vi "configuration UI.vi"() -> ()   [LabVIEW 2013, in "Shared Memory Editor Node.lvclass"]
doc: "Copyright 2016 National Instruments Corporation\n\nLicensed under the Apache License, Version 2.0 (the \"License\"); you may not use this file except in compliance with the License. You may obtain a copy of the License at http://www.apache.org/licenses/LICENSE-2.0\nUnless required by applicable law or agreed to in writing, software distributed under the License is distributed on an \"AS IS\" BASIS, WITHOUT WARRANTIES OR CONDITIONS OF ANY KIND, either express or implied. See the License for the specific language governing permissions and limitations under the License."
uses:
  Shared Memory Editor Node.lvclass
  <vilib>/NI/DCAF UI Toolkit/Controls/Remove.ctl
  <vilib>/NI/DCAF UI Toolkit/Controls/Add.ctl
  <vilib>/NI/Configuration Framework/Node/NodeRef.ctl
  <vilib>/NI/Configuration Framework/Node/NISE_CEF_Node.lvclass
  <vilib>/NI/AMC/Message Queue.ctl
  <vilib>/NI/AMC/Message.ctl
  <vilib>/NI/Tools/Keyed Array/KeyedArray.ctl
  <vilib>/NI/Configuration Framework/Node/UserEventRef.ctl
  <vilib>/NI/Configuration Framework/Controls/EventCluster.ctl
  <vilib>/NI/Configuration Framework/Node/StopEvent.ctl
  <vilib>/NI/Configuration Framework/Node/RefreshUIEvent.ctl
  <vilib>/NI/Configuration Framework/Node/CacheState.ctl
  <vilib>/NI/Configuration Framework/Node/NodeChangeEvent.ctl
  <vilib>/NI/Tag Bus/tag/Data Type.ctl
  <vilib>/NI/DCAF/Tag Editor Core/control module/editor node/channel action event.ctl
  <vilib>/NI/DCAF/Tag Editor Core/control module/editor node/dialog output action.ctl
  <vilib>/NI/Tag Bus Module Framework/channel/TBM channel.lvclass
  <vilib>/NI/Tag Bus/tag/tag descriptor.lvclass
  access.ctl
  <vilib>/NI/DCAF Table API/Table Manager/object ref.ctl
  <vilib>/NI/DCAF/Tag Editor Core/Configuration Editor/Classes/Engine Parent/Engine Parent Editor Node.lvclass
  <vilib>/NI/DCAF/Tag Editor Core/Configuration Editor/Classes/Module editor node/module editor node.lvclass
  <vilib>/NI/DCAF Table API/Table Manager/references.ctl
  <vilib>/NI/DCAF Table API/Listbox/Multi Column Listbox.lvclass
  <vilib>/Utility/miscctls.llb/LVPositionTypeDef.ctl
  <vilib>/NI/DCAF Table API/Listbox/Multi Column Listbox.lvclass/Multi Column Listbox.ctl
  <vilib>/NI/DCAF Table API/Table Manager/Table Manager.lvclass/Table Manager.ctl
  <vilib>/NI/DCAF Table API/Listbox/Write Listbox.vi
  <vilib>/NI/DCAF Table API/Table Manager/Write Top VI.vi
  <vilib>/NI/DCAF/Tag Editor Core/Configuration Editor/Classes/Engine Parent/read engine configuration.vi
  <vilib>/NI/Module Execution Interface/Engine Configuration/engine configuration.lvclass
  <vilib>/NI/DCAF/Tag Editor Core/control module/editor node/control module editor.lvclass
  <vilib>/NI/DCAF Table API/Table Manager/Table Manager.lvclass
  <vilib>/NI/Tools/Keyed Array/Tools_KeyedArray.lvlib
  <vilib>/NI/AMC/AMC.lvlib
  <vilib>/NI/Configuration Framework/NISE_CEF_TreeControl.lvlib
  <vilib>/NI/DCAF UI Toolkit/Controls/DCAF UI Elements.lvlib
panel:
  in  "data type":T1
  in  "access":T2
  in  "Top Level Tab Control":enum32{"<Main Page>", "Configuration"}(tab)
  in  "tag list box":i32(listbox)=1
  in  "remove tag":T3
  in  "Add tag":T4
  in  "write directory":string
  in  "read directory":string
  in  "user event out":refnum<user-event>
  in  "node change":T5
  in  "cache state":T6
  in  "refresh UI":T7
  in  "stop event":T8
  in  "user event":T9
  in  "main queue":T10
  in  "node ref":T11
  # "Directories relative to engine root (/dev/shm/<EngineName>)"
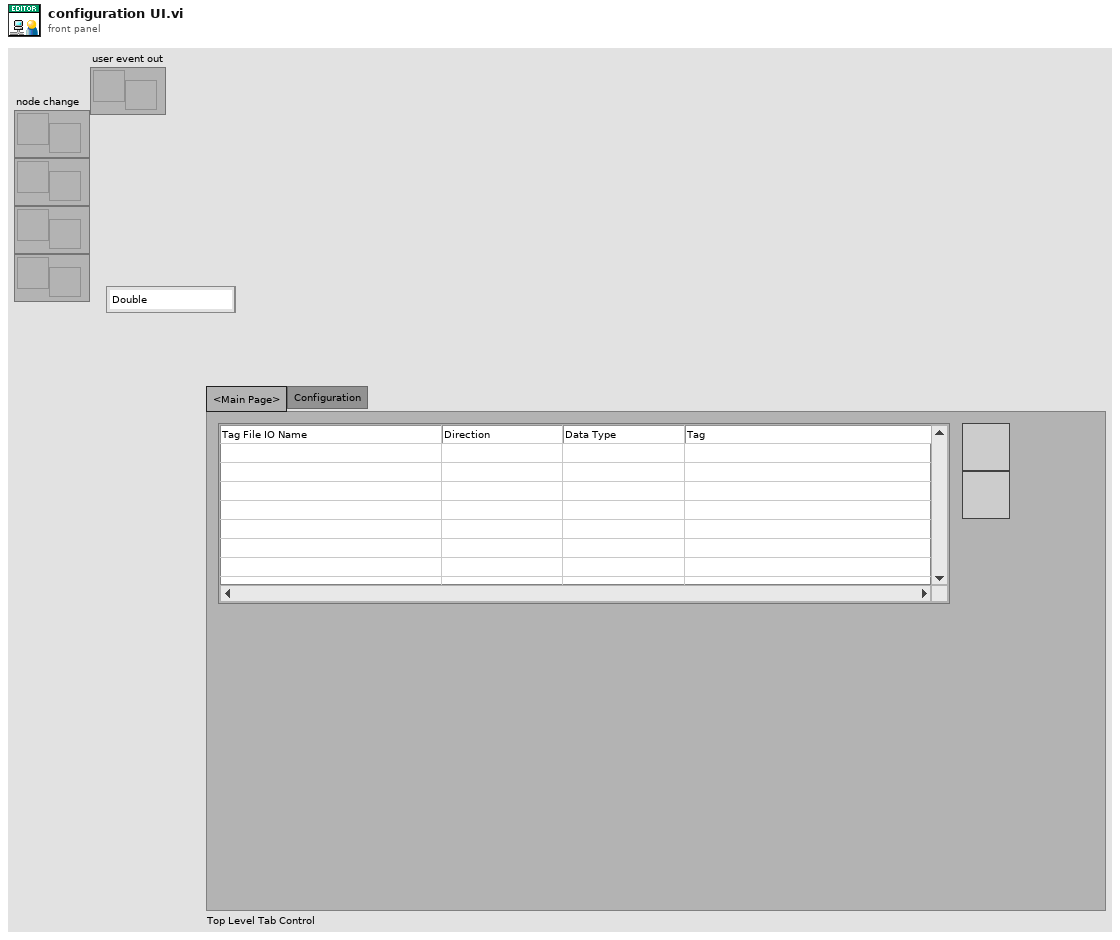
[diagram p1: front panel]
types:
  T1 = typedef "tag bus.lvlib/tag descriptor.lvclass/Data Type.ctl" = enum16{"Double", "Single", "I64", "I32", "I16", "I8", "U64", "U32", "U16", "U8", "Boolean", "String", "Array of Double", "Array of Single", "Array of I64", "Array of I32", "Array of I16", "Array of I8", "Array of U64", "Array of U32", "Array of U16", "Array of U8", "Array of Boolean", "Array of String"}
  T2 = typedef "Shared Memory Editor Node.lvclass/access.ctl" = enum16{"Read from File", "Write to File"}
  T3 = typedef "DCAF UI Elements.lvlib/Remove.ctl" = bool
  T4 = typedef "DCAF UI Elements.lvlib/Add.ctl" = bool
  T5 = typedef "NISE_CEF_Node.lvclass/NodeChangeEvent.ctl" = refnum<user-event>
  T6 = typedef "NISE_CEF_Node.lvclass/CacheState.ctl" = refnum<user-event>
  T7 = typedef "NISE_CEF_Node.lvclass/RefreshUIEvent.ctl" = refnum<user-event>
  T8 = typedef "NISE_CEF_Node.lvclass/StopEvent.ctl" = refnum<user-event>
  T9 = typedef "NISE_CEF_Node.lvclass/UserEventRef.ctl" = refnum<user-event>
  T10 = typedef "AMC.lvlib/Message Queue.ctl" = refnum<queue>
  T11 = typedef "NISE_CEF_Node.lvclass/NodeRef.ctl" = refnum<data-value>
  T12 = typedef "LVPositionTypeDef.ctl" = cluster{"Left":i32, "Top":i32}
  T13 = typedef "Table Manager.lvlib/Table Manager.lvclass/references.ctl" = cluster{"stop event":T8, "refresh UI":T7, "cache state":T6, "node change":T5, "user event out":refnum<user-event>, "main queue":T10, "user event":T9}
  T14 = typedef "Table Manager.lvlib/Table Manager.lvclass/object ref.ctl" = cluster{"engine":refnum<data-value>, "Node Ref":refnum<data-value>}
  T15 = typedef "Table Manager.lvlib/Column.lvclass/Column Descriptor.ctl" = cluster{"name":string, "caption":string, "Column Type":T16, "Params":string, "AutoSizeMode":i32, "FillWeight":sgl, "MinWidth":u32, "tooltip":string, "Enum Reference":refnum<vi>, "Channel suffix":string, "Read Only":bool, "Call Back VI":T17, "DT Dependency":i32, "name dependency":i32, "data type":T1}
  T16 = typedef "Table Manager.lvlib/Column.lvclass/Column Type.ctl" = enum16{"String", "Mapping", "Channel Name", "Tag", "Enum", "Data Type", "Numeric"}
  T17 = typedef "Table Manager.lvlib/Table Manager.lvclass/Call Back Ref Type Def.ctl" = refnum<vi>
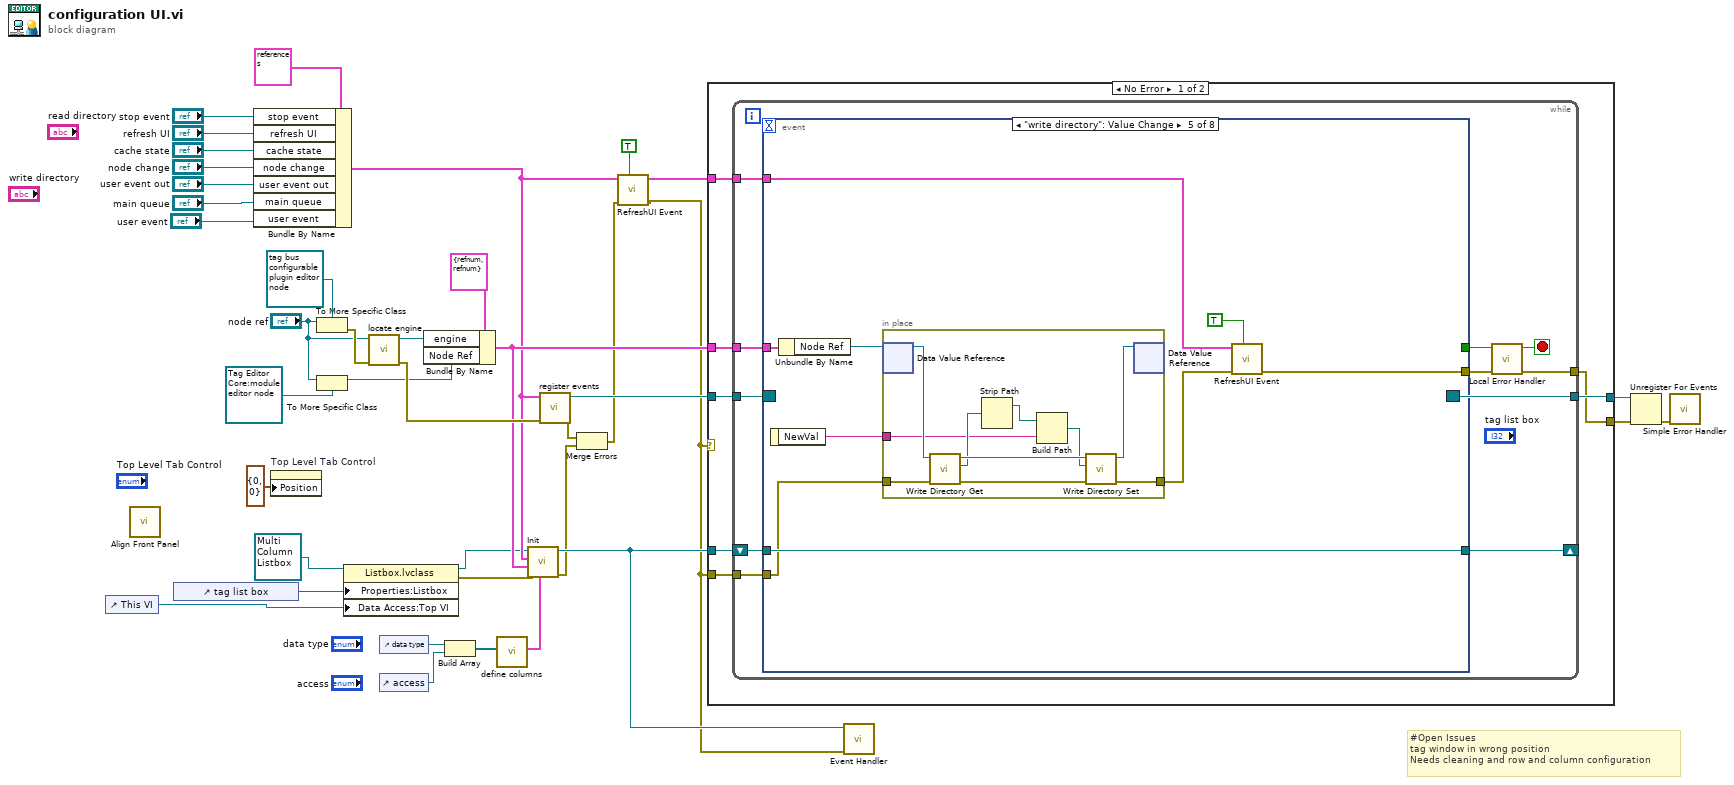
[diagram p0: block diagram]
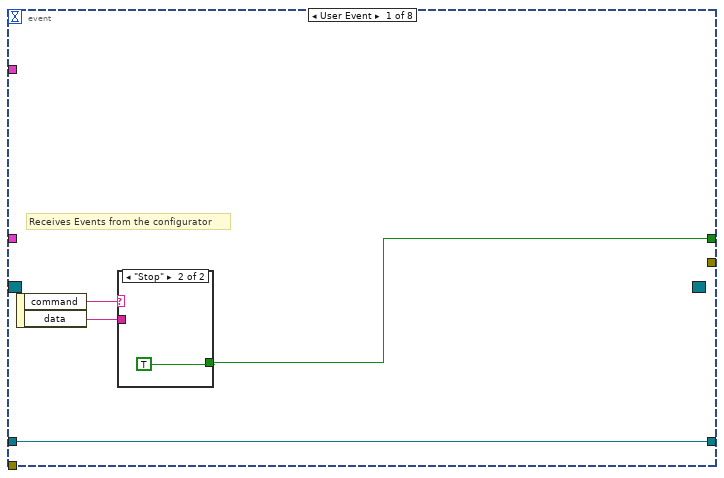
[diagram p2: hidden frame]
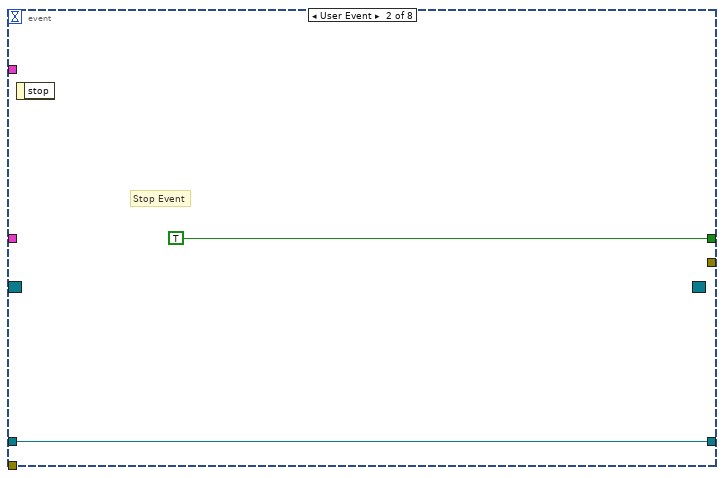
[diagram p4: hidden frame]
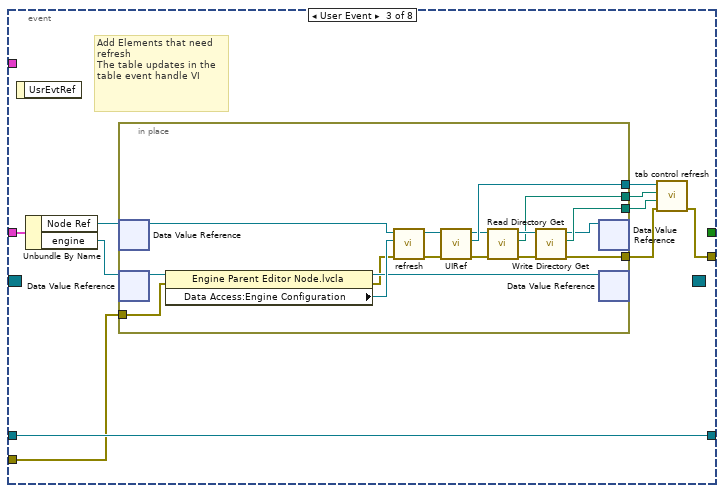
[diagram p5: hidden frame]
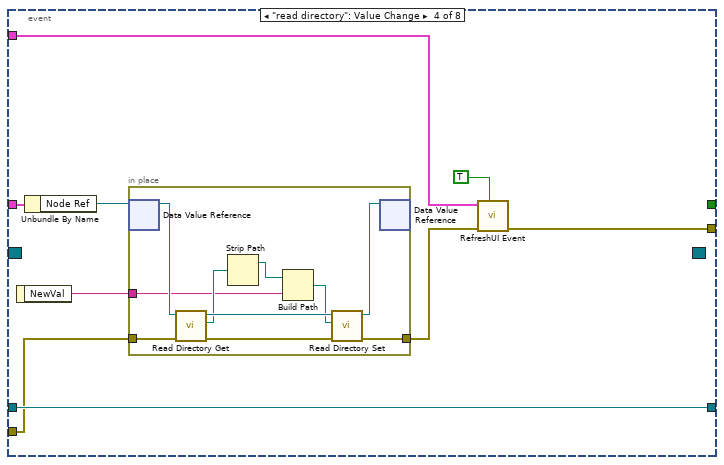
[diagram p6: hidden frame]
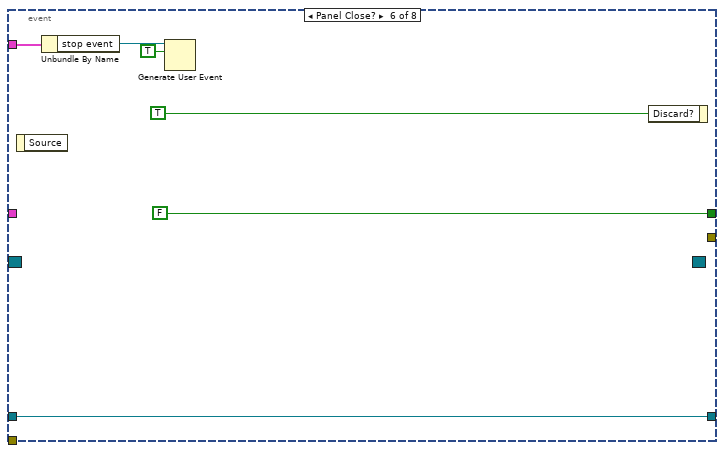
[diagram p7: hidden frame]
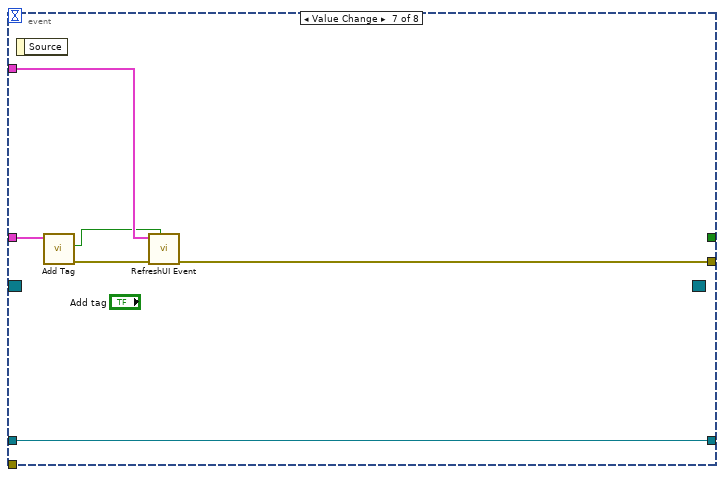
[diagram p8: hidden frame]
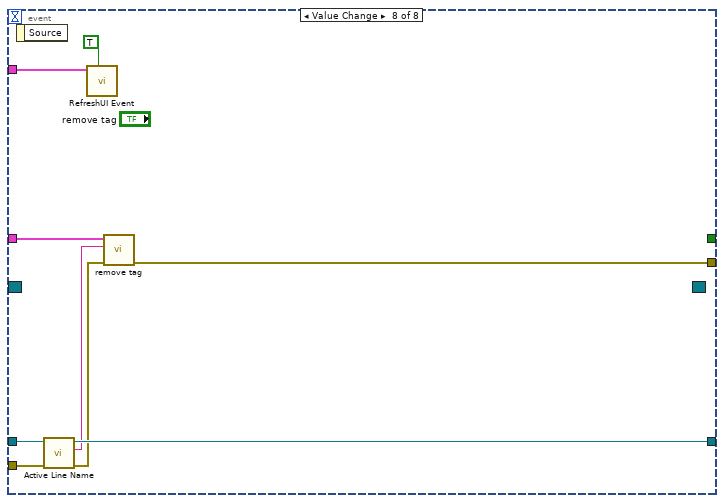
[diagram p9: hidden frame]
diagram:
  # "#Open Issues \ntag window in wrong position\nNeeds cleaning and row and column configuration"
  n1 = control-ref of="This VI"() -> (w17:refnum<vi>)
  n2 = call <vilib>:"Align Front Panel.vi"() -> ()  [unwired: 10 in, 2 out]
  n3 = control-ref of="tag list box"() -> (w18:refnum<vi>)
  n4 = Bundle By Name(cluster=T13 {"stop event"=refnum, "refresh UI"=refnum, "cache state"=refnum, "node change"=refnum, "user event out"=refnum, "main queue"=refnum, "user event"=refnum} ("References"), "stop event"="stop event", "refresh UI"="refresh UI", "cache state"="cache state", "node change"="node change", "user event out"="user event out", "main queue"="main queue", "user event"="user event") -> (w15:T13)
  n5 = property on="Top Level Tab Control" class="TabCtl (strict)"("Position"=T12 {"Left"=0, "Top"=0}) -> ()  [unwired: 2 in, 2 out]
  n6 = To More Specific Class(target class=refnum<data-value> refnum ("data value reference"), reference="node ref") -> (error out=w25:errorcluster)  [unwired: 1 in, 1 out]
  n7 = To More Specific Class(target class=refnum<data-value> refnum ("data value reference"), reference="node ref") -> (specific class reference=w9:refnum<data-value>)  [unwired: 1 in, 1 out]
  n8 = property class="Listbox.lvclass"(reference=refnum<class "Multi Column Listbox.lvclass"> refnum ("Table Manager.lvlib:Multi Column Listbox.lvclass"), "Properties:Listbox"=w18, "Data Access:Top VI"=w17) -> (reference out=w8:refnum<class "Multi Column Listbox.lvclass">, error out=w21:errorcluster)  [unwired: 1 in]
  n9 = call <vilib>:"locate engine.vi"("error in"=w25, "component"="node ref") -> ("error out"=w22:errorcluster, "engine"=w24:refnum<data-value>)  [unwired: 8 in]
  n10 = control-ref of="data type"() -> (w5:refnum<vi>)
  n11 = control-ref of="access"() -> (w7:refnum<vi>)
  n12 = Bundle By Name(cluster=T14 {"engine"=refnum, "Node Ref"=refnum} ("references"), "engine"=w24, "Node Ref"=w9) -> (w16:T14)
  n13 = Build Array(w5, w7) -> (w4:refnum<vi>[])
  n14 = call "define columns.vi"("enum references"=w4) -> ("Column Definition"=w20:T15[])  [unwired: 10 in]
  n15 = call-dynamic "Init.vi"("Column Definitions"=w20, "error in (no error)"=w21, "object refs"=w16, "References in"=w15, "Multi Column Listbox in"=w8) -> ("error out"=w14:errorcluster, "Multi Column Listbox out"=w35:refnum<class "Multi Column Listbox.lvclass">)  [unwired: 4 in, 1 out]
  n16 = call "register events.vi"("error in"=w22, "References"=w15) -> ("error out"=w13:errorcluster, "Event Registration Refnum"=w36:refnum<event-registration>)  [unwired: 8 in]
  n17 = Merge Errors(w13, w14) -> (w12:errorcluster)
  n18 = call "RefreshUI Event.vi"("Refresh?"=TRUE, "error in"=w12, "References in"=w15) -> ("error out"=w2:errorcluster, "References out"=w1:T13)  [unwired: 7 in]
  n19 = case shown="No Error" w2 {
    selector: w2 -> [_ w152]
    tunnel: w36 -> [w46 w151]
    tunnel: [w45 w151] -> w39
    tunnel: [w44 w152] -> w38
    tunnel: w1 -> [w43 _]
    tunnel: w16 -> [w42 _]
    tunnel: w35 -> [w41 _]
    tunnel: w2 -> [w40 _]
    frame No Error {
      n20 = while {
        tunnel: w46 -> [w57]
        tunnel: [w56] -> w45
        tunnel: [w53] -> w44
        tunnel: w43 -> [w51]
        tunnel: w42 -> [w50]
        shift-right: [w48] -> _
        shift-left: w41 -> [w49]
        tunnel: w40 -> [w47]
        stop <- w55 stop-if-true
        n21 = event shown="[4] \"write directory\": Value Change" {
          selector: w57 -> [_ _ _ _ _ _ _ _]
          dyn-events: [_ _ _ _ _ _ _ _] -> w56
          timeout: _ -> [_ _ _ _ _ _ _ _]
          tunnel: [w61 TRUE _ _ _ FALSE _ _] -> w54
          tunnel: [_ _ w65 w94 w113 _ w137 w150] -> w52
          tunnel: w51 -> [_ _ _ w96 w115 w131 w140 w148]
          tunnel: w50 -> [_ _ w72 w99 w118 _ w136 w147]
          tunnel: w49 -> [w58 w63 w74 w100 w119 w130 w141 w146]
          tunnel: [w58 w63 w74 w100 w119 w130 w141 w144] -> w48
          tunnel: w47 -> [_ _ w73 w97 w116 _ _ w145]
          event User Event {
            # "Receives Events from the configurator"
            n22 = event-data() -> ("command"=w60:string, "data"=w59:string)  [unwired: 1 in]
            n23 = case shown="\"Stop\"" w60 {
              tunnel: [_ TRUE] -> w61
              tunnel: w59 -> [_ _]
              frame Default {
              }
              frame "Stop" {
              }
            }
          }
          event User Event {
            # "Stop Event"
            n24 = event-data() -> ()  [unwired: 1 in, 1 out]
          }
          event User Event {
            # "Add Elements that need refresh \nThe table updates in the table event handle VI"
            n25 = event-data() -> ()  [unwired: 1 in, 1 out]
            n26 = Unbundle By Name(w72) -> ("Node Ref"=w71:refnum<data-value>, "engine"=w70:refnum<data-value>)
            n27 = in-place {
              in-place-border: w73 -> [w88]
              in-place-border: [w80] -> w66
              in-place-border: [w84] -> w68
              in-place-border: [w83] -> w67
              in-place-border: [w82] -> w69
              n28 = in-place-dvr #1(w71) -> (w75:refnum<class "module editor node.lvclass">)  [unwired: 1 out]
              n29 = in-place-dvr #2(w70) -> (w91:refnum<class "Engine Parent Editor Node.lvclass">)  [unwired: 1 out]
              n30 = property class="Engine Parent Editor Node.lvcla"(reference=w91, error in=w88) -> (reference out=w89:refnum<class "Engine Parent Editor Node.lvclass">, error out=w87:errorcluster, "Data Access:Engine Configuration"=w90:refnum<class "engine configuration.lvclass">)
              n31 = call-dynamic "refresh.vi"("error in (no error)"=w87, "Engine Configuration In"=w90, "Module Editor Node In"=w75) -> ("error out"=w77:errorcluster, "Module Editor Node Out"=w79:refnum<class "module editor node.lvclass">)  [unwired: 6 in, 1 out]
              n32 = call-dynamic "UIRef.vi"("error in"=w77, "node in"=w79) -> ("error out"=w76:errorcluster, "VI refnum"=w82:refnum<vi>, "node out"=w78:refnum<class "module editor node.lvclass">)  [unwired: 7 in]
              n33 = call "Read Directory Get.vi"("error in"=w76, "node"=w78) -> ("error out"=w85:errorcluster, "file directory"=w84:path, "node out"=w86:refnum<class "module editor node.lvclass">)  [unwired: 7 in]
              n34 = call "Write Directory Get.vi"("error in"=w85, "node"=w86) -> ("error out"=w80:errorcluster, "file directory"=w83:path, "node out"=w81:refnum<class "module editor node.lvclass">)  [unwired: 7 in]
              n35 = in-place-dvr #1(w81) -> ()  [unwired: 2 out]
              n36 = in-place-dvr #2(w89) -> ()  [unwired: 2 out]
            }
            n37 = call "tab control refresh.vi"("error in"=w66, "write directory"=w67, "read directory"=w68, "VI reference"=w69) -> ("error out"=w65:errorcluster)  [unwired: 7 in]
          }
          event "read directory": Value Change {
            n38 = event-data() -> ("NewVal"=w92:string)  [unwired: 1 in]
            n39 = Unbundle By Name(w99) -> ("Node Ref"=w98:refnum<data-value>)
            n40 = in-place {
              in-place-border: w97 -> [w107]
              in-place-border: [w109] -> w95
              in-place-border: w92 -> [w102]
              n41 = in-place-dvr #3(w98) -> (w108:refnum<class "module editor node.lvclass">)  [unwired: 1 out]
              n42 = call "Read Directory Get.vi"("error in"=w107, "node"=w108) -> ("error out"=w106:errorcluster, "file directory"=w104:path, "node out"=w105:refnum<class "module editor node.lvclass">)  [unwired: 7 in]
              n43 = Strip Path(path=w104) -> (stripped path=w103:path)  [unwired: 1 out]
              n44 = Build Path(base path=w103, name or relative path=w102) -> (appended path=w101:path)
              n45 = call "Read Directory Set.vi"("error in"=w106, "file directory"=w101, "node"=w105) -> ("error out"=w109:errorcluster, "node out"=w110:refnum<class "module editor node.lvclass">)  [unwired: 7 in]
              n46 = in-place-dvr #3(w110) -> ()  [unwired: 2 out]
            }
            n47 = call "RefreshUI Event.vi"("Refresh?"=TRUE, "error in"=w95, "References in"=w96) -> ("error out"=w94:errorcluster)  [unwired: 7 in, 1 out]
          }
          event "write directory": Value Change {
            n48 = event-data() -> ("NewVal"=w111:string)  [unwired: 1 in]
            n49 = Unbundle By Name(w118) -> ("Node Ref"=w117:refnum<data-value>)
            n50 = in-place {
              in-place-border: w116 -> [w126]
              in-place-border: [w128] -> w114
              in-place-border: w111 -> [w121]
              n51 = in-place-dvr #4(w117) -> (w127:refnum<class "module editor node.lvclass">)  [unwired: 1 out]
              n52 = call "Write Directory Get.vi"("error in"=w126, "node"=w127) -> ("error out"=w125:errorcluster, "file directory"=w123:path, "node out"=w124:refnum<class "module editor node.lvclass">)  [unwired: 7 in]
              n53 = Strip Path(path=w123) -> (stripped path=w122:path)  [unwired: 1 out]
              n54 = Build Path(base path=w122, name or relative path=w121) -> (appended path=w120:path)
              n55 = call "Write Directory Set.vi"("error in"=w125, "file directory"=w120, "node"=w124) -> ("error out"=w128:errorcluster, "node out"=w129:refnum<class "module editor node.lvclass">)  [unwired: 7 in]
              n56 = in-place-dvr #4(w129) -> ()  [unwired: 2 out]
            }
            n57 = call "RefreshUI Event.vi"("Refresh?"=TRUE, "error in"=w114, "References in"=w115) -> ("error out"=w113:errorcluster)  [unwired: 7 in, 1 out]
          }
          event Panel Close? {
            n58 = event-data() -> ()  [unwired: 1 in, 1 out]
            n59 = Unbundle By Name(w131) -> ("stop event"=w132:T8)
            n60 = Generate User Event(user event=w132, event data cluster=TRUE ("event data")) -> ()  [unwired: 2 in, 2 out]
            n61 = event-data("Discard?"=TRUE) -> ()  [unwired: 1 in, 1 out]
          }
          event Value Change {
            n62 = event-data() -> ()  [unwired: 1 in, 1 out]
            n63 = call "Add Tag.vi"("references"=w136) -> ("error out"=w138:errorcluster, "newtag?"=w139:bool)  [unwired: 9 in]
            n64 = call "RefreshUI Event.vi"("Refresh?"=w139, "error in"=w138, "References in"=w140) -> ("error out"=w137:errorcluster)  [unwired: 7 in, 1 out]
          }
          event Value Change {
            n65 = event-data() -> ()  [unwired: 1 in, 1 out]
            n66 = call-dynamic "Active Line Name.vi"("error in"=w145, "Multi Column Listbox in"=w146) -> ("error out"=w142:errorcluster, "Active Line Name"=w143:string, "Multi Column Listbox out"=w144:refnum<class "Multi Column Listbox.lvclass">)  [unwired: 7 in]
            n67 = call "RefreshUI Event.vi"("Refresh?"=TRUE, "References in"=w148) -> ()  [unwired: 8 in, 2 out]
            n68 = call "remove tag.vi"("error in"=w142, "tag"=w143, "object ref in"=w147) -> ("error out"=w150:errorcluster)  [unwired: 8 in]
          }
        }
        n69 = call "Local Error Handler.vi"("error in"=w52, "stop in"=w54) -> ("error out"=w53:errorcluster, "stop out"=w55:bool)  [unwired: 8 in]
      }
    }
    frame Error {
    }
  }
  n70 = call-dynamic "Event Handler.vi"("error in"=w2, "Listbox in"=w35) -> ()  [unwired: 8 in, 2 out]
  n71 = Unregister For Events(event registration refnum=w39, error in=w38) -> (error out=w37:errorcluster)
  n72 = call <vilib>:"Simple Error Handler.vi"("error in (no error)"=w37) -> ()  [unwired: 4 in, 5 out]
